vi "lanelog.vi"() -> ()   [LabVIEW 2012]
uses:
  G_VEH.vi
  G_SEN.vi
  G_NAV.vi
  G_PATH.vi
  <vilib>/Analysis/NI_AALBase.lvlib
panel:
  out "Histogram Graph":T1(graph)
  out "Numeric":dbl
  out "Waveform Chart 9":i16(graph)
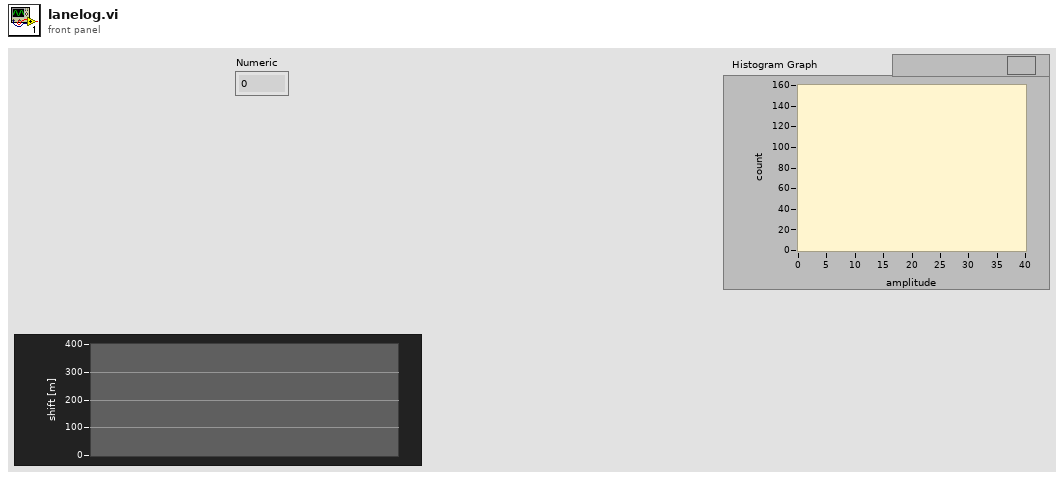
[diagram p1: front panel]
types:
  T1 = cluster{"X Values":dbl[], "Histogram: h(x)":i32[]}
  T2 = cluster{"idx":i32, "x":dbl, "y":dbl, "h":dbl, "x_path":dbl}
  T3 = cluster{"Steer_input":dbl, "Steer_output":dbl, "VS_des":dbl, "VS_can":dbl, "heading":dbl, "auto":bool, "run":bool, "x":dbl, "y":dbl}
  T4 = cluster{i16, "Real Matrix Element":dbl, "Real Matrix Element":dbl, "element":dbl, "element":dbl}[]
  T5 = cluster{"GPSTime":dbl, "attitude[2]":dbl, "lcc[0]":dbl, "lcc[1]":dbl, "heading_GPS":dbl}
  T6 = cluster{"Real Matrix Element":i16, "Real Matrix Element":dbl}[]
  T7 = cluster{"idx":dbl, "x":dbl, "y":dbl, "h":dbl, "x_path":dbl}
  T8 = cluster{i16, "element":dbl, "element":dbl, "element":dbl, "element":dbl}[]
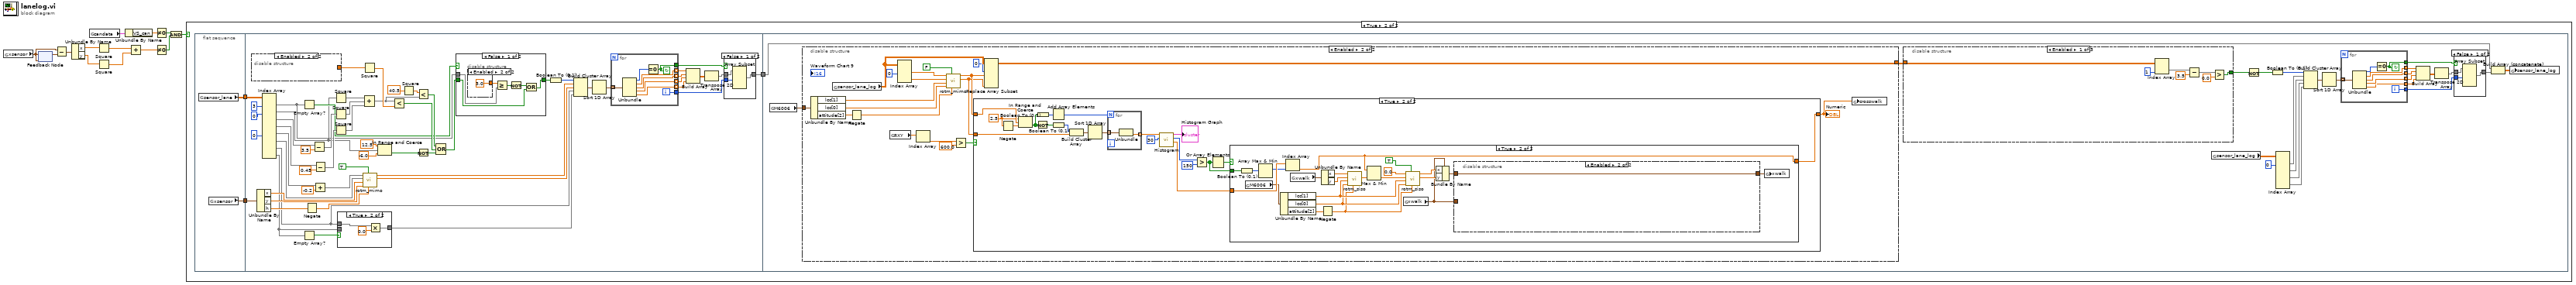
[diagram p0: block diagram]
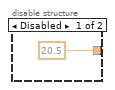
[diagram p3: hidden frame]
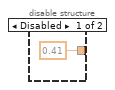
[diagram p5: hidden frame]
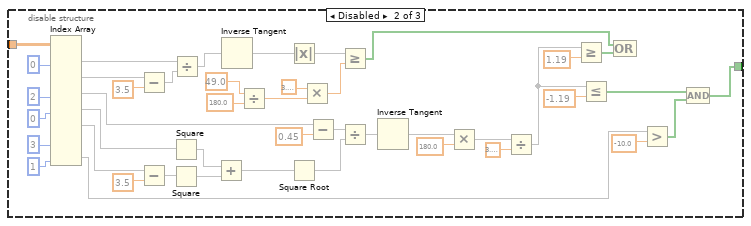
[diagram p8: hidden frame]
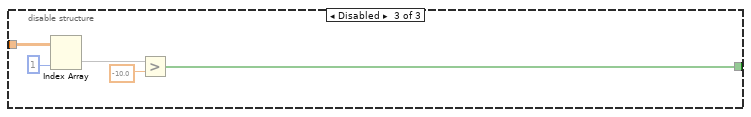
[diagram p9: hidden frame]
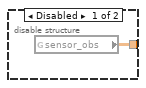
[diagram p11: hidden frame]
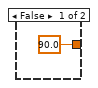
[diagram p12: hidden frame]
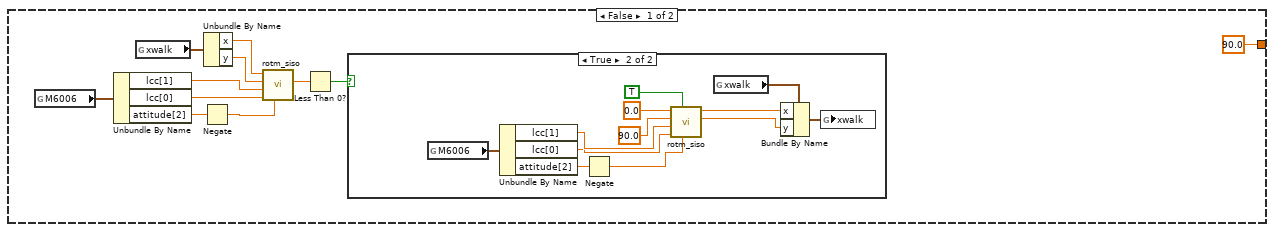
[diagram p13: hidden frame]
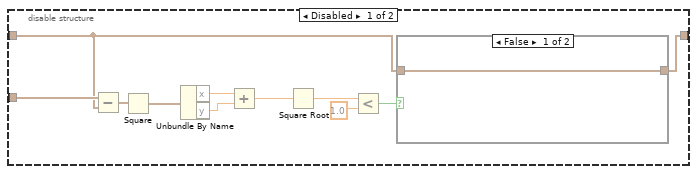
[diagram p15: hidden frame]
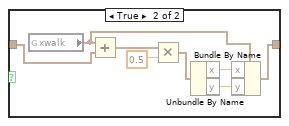
[diagram p16: hidden frame]
diagram:
  n1 = global read "G_VEH.vi" "xsensor"() -> (w1:T2)
  n2 = feedback-in #1(w1) -> ()
  n3 = feedback #1(w1) -> (w11:T2)
  n4 = Subtract(x=w1, y=w11) -> (x-y=w10:T2)
  n5 = Unbundle By Name(w10) -> ("x"=w9:dbl, "y"=w8:dbl)
  n6 = global read "G_VEH.vi" "candata"() -> (w13:T3)
  n7 = Square(x=w9) -> (x^2=w7:dbl)
  n8 = Square(x=w8) -> (x^2=w6:dbl)
  n9 = Unbundle By Name(w13) -> ("VS_can"=w12:dbl)
  n10 = Add(x=w7, y=w6) -> (x+y=w5:dbl)
  n11 = Not Equal To 0?(x=w12) -> (x != 0?=w3:bool)
  n12 = Not Equal To 0?(x=w5) -> (x != 0?=w4:bool)
  n13 = And(x=w3, y=w4) -> (x .and. y?=w2:bool)
  n14 = case shown="True" w2 {
    frame False {
    }
    frame True {
      n15 = flat-sequence {
        tunnel: [w18] -> w16
        tunnel: [w17] -> w15
        tunnel: [w57] -> w14
        tunnel: w16 -> [w56]
        tunnel: w15 -> [w55]
        tunnel: w14 -> [w104]
        frame #0 {
          n16 = global read "G_SEN.vi" "sensor_lane"() -> (w18:dbl[][])
          n17 = global read "G_VEH.vi" "xsensor"() -> (w17:T2)
        }
        frame #1 {
          n18 = disable-structure shown="Enabled" {
            disable-tunnel: [20.5 ("R 2") _] -> w38
            frame Disabled {
            }
            frame Enabled {
            }
          }
          n19 = Unbundle By Name(w55) -> ("x"=w51:dbl, "y"=w50:dbl, "h"=w49:dbl)
          n20 = Index Array(array=w56, index (col) #1=3 ("disabled index (col)"), index (col) #2=0 ("disabled index (col)"), index (col) #5=0 ("index (col)")) -> (element #1=w34:dbl[], element #2=w26:dbl[], element #3=w44:dbl[], element #4=w42:dbl[], element #5=w21:dbl[], element #6=w54:dbl[], element #7=w27:dbl[], element #8=w28:dbl[])  [unwired: 13 in]
          n21 = Empty Array?(array=w34) -> (empty?=w33:bool)
          n22 = Empty Array?(array=w28) -> (empty?=w30:bool)
          n23 = Negate(x=w49) -> (-x=w48:dbl)
          n24 = Subtract(x=w44, y=3.5) -> (x-y=w43:dbl[])
          n25 = Add(x=w21, y=-0.2) -> (x+y=w20:dbl[])
          n26 = Subtract(x=w42, y=0.45) -> (x-y=w41:dbl[])
          n27 = Square(x=w26) -> (x^2=w74:dbl[])
          n28 = Square(x=w43) -> (x^2=w73:dbl[])
          n29 = Square(x=w41) -> (x^2=w72:dbl[])
          n30 = case shown="True" w30 {
            tunnel: [w77 w79] -> w29
            tunnel: w28 -> [w77 _]
            tunnel: w27 -> [_ w80]
            frame False {
            }
            frame True {
              n31 = Multiply(x=w80, y=0.0) -> (x*y=w79:dbl[])
            }
          }
          n32 = Square(x=w38) -> (x^2=w37:dbl)
          n33 = call "rotm_mimo.vi"("angle[rad]"=w48, "reverse"=TRUE, "y0"=w50, "x0"=w51, "y"=w54, "x"=w20) -> ("Y"=w52:dbl[], "X"=w53:dbl[])  [unwired: 2 in, 2 out]
          n34 = Compound Arithmetic op=ADD(w74, w73, w72) -> (w36:dbl[])
          n35 = In Range and Coerce(upper limit=12.5, x=w26, lower limit=-6.0) -> (In Range?=w25:bool[])  [unwired: 1 out]
          n36 = Less?(x=w36, y=w37) -> (x < y?=w35:bool[])
          n37 = Square(x=40.5 ("R")) -> (x^2=w70:dbl)
          n38 = Less?(x=w70, y=w36) -> (x < y?=w39:bool[])
          n39 = Not(x=w25) -> (.not. x?=w24:bool[])
          n40 = Compound Arithmetic op=OR(w39, w35, w24) -> (w32:bool[])
          n41 = case shown="False" w33 {
            tunnel: w34 -> [w84 _]
            tunnel: w32 -> [w82 w89]
            tunnel: [w81 w89] -> w31
            frame False {
              n42 = disable-structure shown="Enabled" {
                disable-tunnel: [0.41 3.0] -> w85
                frame Disabled {
                }
                frame Enabled {
                }
              }
              n43 = Greater Or Equal?(x=w85, y=w84) -> (x >= y?=w86:bool[])
              n44 = Not(x=w86) -> (.not. x?=w83:bool[])
              n45 = Compound Arithmetic op=OR(w83, w82) -> (w81:bool[])
            }
            frame True {
            }
          }
          n46 = Boolean To (0,1)(Boolean=w31) -> (0, 1=w69:i16[])
          n47 = Build Cluster Array(w69, w53, w52, w27, w29) -> (w67:T4)
          n48 = Sort 1D Array(array=w67) -> (sorted array=w62:T4)
          n49 = for {
            tunnel: w62 -> [w101] mode=indexing
            tunnel: [w100] -> w66 mode=indexing
            tunnel: [w99] -> w65 mode=indexing
            tunnel: [w98] -> w64 mode=indexing
            tunnel: [w97] -> w63 mode=indexing
            tunnel: [w95] -> w59
            tunnel: [w94] -> w58
            i -> [w94]
            stop <- w95 continue-if-true
            n50 = Unbundle(w101) -> (w96:i16, "Real Matrix Element"=w100:dbl, "Real Matrix Element"=w99:dbl, "element"=w98:dbl, "element"=w97:dbl)
            n51 = Equal To 0?(x=w96) -> (x = 0?=w95:bool)
          }
          n52 = Build Array(w66, w65, w64, w63) -> (w61:dbl[][])
          n53 = Transpose 2D Array(2D array=w61) -> (transposed array=w60:dbl[][])
          n54 = case shown="False" w59 {
            tunnel: w60 -> [w92 w93]
            tunnel: w58 -> [w90 _]
            tunnel: [w91 w93] -> w57
            frame False {
              n55 = Array Subset(array=w92, length (row)=w90) -> (w91:dbl[][])  [unwired: 3 in]
            }
            frame True {
            }
          }
        }
        frame #2 {
          n56 = global read "G_NAV.vi" "M6006"() -> (w102:T5)
          n57 = disable-structure shown="Enabled" {
            disable-tunnel: [w194 w202] -> w108
            disable-tunnel: w102 -> [_ w203]
            frame Disabled {
              n58 = global read "G_SEN.vi" "sensor_obs"() -> (w194:dbl[][])
            }
            frame Enabled {
              n59 = Unbundle By Name(w203) -> ("lcc[1]"=w210:dbl, "lcc[0]"=w209:dbl, "attitude[2]"=w208:dbl)
              n60 = global read "G_SEN.vi" "sensor_lane_log"() -> (w205:dbl[][])
              n61 = Negate(x=w208) -> (-x=w207:dbl)
              n62 = global read "G_PATH.vi" "RXY"() -> (w199:dbl[])
              n63 = Index Array(array=w205, index (col) #1=0 ("disabled index (col)")) -> (element #1=w212:dbl[], element #2=w211:dbl[])  [unwired: 3 in]
              n64 = Index Array(array=w199) -> (element=w198:dbl)  [unwired: 1 in]
              n65 = call "rotm_mimo.vi"("angle[rad]"=w207, "reverse"=FALSE, "y0"=w209, "x0"=w210, "y"=w211, "x"=w212) -> ("Y"=w200:dbl[], "X"=w201:dbl[])  [unwired: 2 in, 2 out]
              n66 = Greater?(x=w198, y=600.0) -> (0:w196:bool)
              n67 = case shown="True" w196 {
                tunnel: w201 -> [_ w234]
                tunnel: w200 -> [_ w228]
                tunnel: [90.0 w217] -> w195
                frame False {
                }
                frame True {
                  w232 = 2.5
                  n68 = Negate(x=w232) -> (-x=w233:dbl)
                  n69 = In Range and Coerce(upper limit=w232, x=w234, lower limit=w233) -> (In Range?=w227:bool[])  [unwired: 1 out]
                  n70 = Boolean To (0,1)(Boolean=w227) -> (0, 1=w226:i16[])
                  n71 = Not(x=w227) -> (.not. x?=w230:bool[])
                  n72 = Add Array Elements(numeric array=w226) -> (sum=w216:i16)
                  n73 = Boolean To (0,1)(Boolean=w230) -> (0, 1=w229:i16[])
                  n74 = Build Cluster Array(w229, w228) -> (w225:T6)
                  n75 = Sort 1D Array(array=w225) -> (sorted array=w224:T6)
                  n76 = for {
                    N: w216 -> [_]
                    tunnel: w224 -> [w236] mode=indexing
                    tunnel: [w235] -> w223 mode=indexing
                    n77 = Unbundle(w236) -> ("Real Matrix Element"=w235:dbl)  [unwired: 1 out]
                  }
                  n78 = call <vilib>:"Histogram.vi"("intervals"=30, "X"=w223) -> ("X Values"=w218:dbl[], "Histogram: h(x)"=w222:i32[], "Histogram Graph"=→"Histogram Graph":T1)  [unwired: 6 in, 1 out]
                  n79 = Greater?(x=w222, y=150) -> (0:w219:bool[])
                  n80 = Or Array Elements(Boolean array=w219) -> (logical OR=w220:bool)
                  n81 = case shown="True" w220 {
                    tunnel: w219 -> [_ w281]
                    tunnel: w218 -> [_ w279]
                    tunnel: [90.0 w264] -> w217
                    frame False {
                      n82 = global read "G_NAV.vi" "M6006"() -> (w245:T5)
                      n83 = Unbundle By Name(w245) -> ("lcc[1]"=w242:dbl, "lcc[0]"=w243:dbl, "attitude[2]"=w246:dbl)
                      n84 = global read "G_VEH.vi" "xwalk"() -> (w241:T2)
                      n85 = Negate(x=w246) -> (-x=w244:dbl)
                      n86 = Unbundle By Name(w241) -> ("x"=w240:dbl, "y"=w239:dbl)
                      n87 = call "rotm_siso.vi"("angle[rad]"=w244, "y0"=w243, "x0"=w242, "y"=w239, "x"=w240) -> ("y'"=w238:dbl)  [unwired: 5 in, 1 out]
                      n88 = Less Than 0?(x=w238) -> (x < 0?=w237:bool)
                      n89 = case shown="True" w237 {
                        frame False {
                        }
                        frame True {
                          n90 = global read "G_NAV.vi" "M6006"() -> (w256:T5)
                          n91 = Unbundle By Name(w256) -> ("lcc[1]"=w259:dbl, "lcc[0]"=w258:dbl, "attitude[2]"=w255:dbl)
                          n92 = Negate(x=w255) -> (-x=w257:dbl)
                          n93 = call "rotm_siso.vi"("angle[rad]"=w257, "reverse"=TRUE, "y0"=w258, "x0"=w259, "y"=90.0, "x"=0.0) -> ("y'"=w249:dbl, "x'"=w250:dbl)  [unwired: 4 in]
                          n94 = global read "G_VEH.vi" "xwalk"() -> (w251:T2)
                          n95 = Bundle By Name(cluster=w251, "x"=w250, "y"=w249) -> (w248:T2)
                          n96 = global write "G_VEH.vi" "xwalk"(w248) -> ()
                        }
                      }
                    }
                    frame True {
                      n97 = Boolean To (0,1)(Boolean=w281) -> (0, 1=w280:i16[])
                      n98 = global read "G_NAV.vi" "M6006"() -> (w276:T5)
                      n99 = Array Max & Min(array=w280) -> (max index (indices)=w278:i32)  [unwired: 3 out]
                      n100 = Unbundle By Name(w276) -> ("lcc[1]"=w262:dbl, "lcc[0]"=w261:dbl, "attitude[2]"=w277:dbl)
                      n101 = Index Array(array=w279, index=w278) -> (element=w264:dbl)
                      n102 = global read "G_VEH.vi" "xwalk"() -> (w268:T2)
                      n103 = Negate(x=w277) -> (-x=w260:dbl)
                      n104 = Unbundle By Name(w268) -> ("x"=w267:dbl, "y"=w266:dbl)
                      n105 = call "rotm_siso.vi"("angle[rad]"=w260, "y0"=w261, "x0"=w262, "y"=w266, "x"=w267) -> ("y'"=w265:dbl)  [unwired: 5 in, 1 out]
                      n106 = Max & Min(x=w264, y=w265) -> (min(x,y)=w263:dbl)  [unwired: 1 out]
                      n107 = global read "G_VEH.vi" "xwalk"() -> (w271:T2)
                      n108 = call "rotm_siso.vi"("angle[rad]"=w260, "reverse"=TRUE, "y0"=w261, "x0"=w262, "y"=w263, "x"=0.0) -> ("y'"=w272:dbl, "x'"=w273:dbl)  [unwired: 4 in]
                      n109 = Bundle By Name(cluster=w271, "x"=w273, "y"=w272) -> (w269:T2)
                      n110 = disable-structure shown="Enabled" {
                        disable-tunnel: w271 -> [w292 _]
                        disable-tunnel: [w283 w302] -> w270
                        disable-tunnel: w269 -> [w282 w302]
                        frame Disabled {
                          n111 = Subtract(x=w292, y=w282) -> (x-y=w291:T2)
                          n112 = Square(x=w291) -> (x^2=w290:T2)
                          n113 = Unbundle By Name(w290) -> ("x"=w288:dbl, "y"=w289:dbl)
                          n114 = Add(x=w288, y=w289) -> (x+y=w287:dbl)
                          n115 = Square Root(x=w287) -> (sqrt(x)=w286:dbl)
                          n116 = Less?(x=w286, y=1.0) -> (x < y?=w284:bool)
                          n117 = case shown="False" w284 {
                            tunnel: [w293 w297] -> w283
                            tunnel: w282 -> [w293 w301]
                            frame False {
                            }
                            frame True {
                              n118 = global read "G_VEH.vi" "xwalk"() -> (w298:T2)
                              n119 = Add(x=w298, y=w301) -> (x+y=w300:T2)
                              n120 = Multiply(x=w300, y=0.5) -> (x*y=w296:T7)
                              n121 = Unbundle By Name(w296) -> ("x"=w295:dbl, "y"=w294:dbl)
                              n122 = Bundle By Name(cluster=w298, "x"=w295, "y"=w294) -> (w297:T2)
                            }
                          }
                        }
                        frame Enabled {
                        }
                      }
                      n123 = global write "G_VEH.vi" "xwalk"(w270) -> ()
                    }
                  }
                }
              }
              "Numeric" <- w195
              n124 = Replace Array Subset(array=w205, new element #1=w201, index (col) #1=0 ("disabled index (col)"), new element #2=w200) -> (w202:dbl[][])  [unwired: 3 in]
              n125 = global write "G_SEN.vi" "crosswalk"(w195) -> ()
            }
          }
          n126 = disable-structure shown="Enabled" {
            disable-tunnel: w108 -> [w131 w143 w181]
            disable-tunnel: [w130 w142 w177] -> w107
            frame Enabled {
              n127 = Index Array(array=w131, index (col)=1) -> (element=w128:dbl[])  [unwired: 1 in]
              n128 = Subtract(x=w128, y=3.5) -> (x-y=w127:dbl[])
              n129 = Greater?(x=w127, y=0.0) -> (0:w130:bool[])
            }
            frame Disabled {
              n130 = Index Array(array=w143, index (col) #1=0 ("disabled index (col)"), index (col) #3=2 ("disabled index (col)"), index (col) #4=0 ("disabled index (col)"), index (col) #6=3 ("index (col)"), index (col) #7=1 ("index (col)")) -> (element #1=w156:dbl[], element #2=w141:dbl[], element #3=w168:dbl[], element #4=w158:dbl[], element #5=w174:dbl[], element #7=w146:dbl[])  [unwired: 9 in, 1 out]
              n131 = Subtract(x=w141, y=3.5) -> (x-y=w140:dbl[])
              n132 = Subtract(x=w174, y=3.5) -> (x-y=w159:dbl[])
              n133 = Square(x=w158) -> (x^2=w172:dbl[])
              n134 = Square(x=w159) -> (x^2=w171:dbl[])
              n135 = Divide(x=w156, y=w140) -> (x/y=w155:dbl[])
              n136 = Add(x=w172, y=w171) -> (x+y=w170:dbl[])
              n137 = Inverse Tangent(1:w155) -> (0:w154:dbl[])
              n138 = Divide(x=49.0, y=180.0) -> (x/y=w149:dbl)
              n139 = Absolute Value(x=w154) -> (abs(x)=w153:dbl[])
              n140 = Square Root(x=w170) -> (sqrt(x)=w166:dbl[])
              n141 = Multiply(x=3.141592653589793, y=w149) -> (x*y=w148:dbl)
              n142 = Subtract(x=w168, y=0.45) -> (x-y=w167:dbl[])
              n143 = Greater Or Equal?(x=w153, y=w148) -> (x >= y?=w138:bool[])
              n144 = Divide(x=w167, y=w166) -> (x/y=w165:dbl[])
              n145 = Inverse Tangent(1:w165) -> (0:w161:dbl[])
              n146 = Multiply(x=w161, y=180.0) -> (x*y=w163:dbl[])
              n147 = Divide(x=w163, y=3.141592653589793) -> (x/y=w135:dbl[])
              n148 = Greater Or Equal?(x=w135, y=1.19) -> (x >= y?=w134:bool[])
              n149 = Less Or Equal?(x=w135, y=-1.19) -> (x <= y?=w133:bool[])
              n150 = Compound Arithmetic op=OR(w138, w134) -> ()  [unwired: 1 out]
              n151 = Greater?(x=w146, y=-10.0) -> (0:w144:bool[])
              n152 = Compound Arithmetic op=AND(w133, w144) -> (w142:bool[])
            }
            frame Disabled {
              n153 = Index Array(array=w181, index (col)=1 ("disabled index (col)")) -> (element=w179:dbl[])  [unwired: 1 in]
              n154 = Greater?(x=w179, y=-10.0) -> (0:w177:bool[])
            }
          }
          n155 = global read "G_SEN.vi" "sensor_lane_log"() -> (w103:dbl[][])
          n156 = Not(x=w107) -> (.not. x?=w109:bool[])
          n157 = Boolean To (0,1)(Boolean=w109) -> (0, 1=w124:i16[])
          n158 = Index Array(array=w103, index (col) #1=0 ("disabled index (col)")) -> (element #1=w122:dbl[], element #2=w121:dbl[], element #3=w120:dbl[], element #4=w119:dbl[])  [unwired: 7 in]
          n159 = Build Cluster Array(w124, w122, w121, w120, w119) -> (w125:T8)
          n160 = Sort 1D Array(array=w125) -> (sorted array=w110:T8)
          n161 = for {
            tunnel: w110 -> [w193] mode=indexing
            tunnel: [w192] -> w111 mode=indexing
            tunnel: [w191] -> w112 mode=indexing
            tunnel: [w190] -> w113 mode=indexing
            tunnel: [w189] -> w114 mode=indexing
            tunnel: [w187] -> w117
            tunnel: [w186] -> w118
            i -> [w186]
            stop <- w187 continue-if-true
            n162 = Unbundle(w193) -> (w188:i16, "element"=w192:dbl, "element"=w191:dbl, "element"=w190:dbl, "element"=w189:dbl)
            n163 = Equal To 0?(x=w188) -> (x = 0?=w187:bool)
          }
          n164 = Build Array(w111, w112, w113, w114) -> (w115:dbl[][])
          n165 = Transpose 2D Array(2D array=w115) -> (transposed array=w116:dbl[][])
          n166 = case shown="False" w117 {
            tunnel: w116 -> [w184 w185]
            tunnel: w118 -> [w182 _]
            tunnel: [w183 w185] -> w106
            frame False {
              n167 = Array Subset(array=w184, length (row)=w182) -> (w183:dbl[][])  [unwired: 3 in]
            }
            frame True {
            }
          }
          n168 = Build Array (concatenate)(w104, w106) -> (w105:dbl[][])
          n169 = global write "G_SEN.vi" "sensor_lane_log"(w105) -> ()
        }
      }
    }
  }
